vi "PID Proportional Control start.vi"(0 "Temp":dbl format="%.2f", 7 "Control Parameters":T1={"Setpoint"=50.0, "Control Bandwidth"=4.0, "Integral Time"=30.0, "Int\nON"=TRUE, "Derivative Tme"=0.5, "Der\nON"=TRUE, "Settle Bandwidth"=1.0, "Settle Time"=200.0} {"Settle Time" step=1.0; "Settle Bandwidth" step=0.01; "Derivative Tme" step=0.01; "Integral Time" step=1.0; "Control Bandwidth" step=0.1; "Setpoint" step=0.1}) -> (8 "Proportional Power":dbl format="%.2f")   [LabVIEW 2019]
doc: "Subvi\nThis does the proporianl part of the PID controller \n\nJuan Gamez\nP3600\nCSUSB"
uses:
  typedefs/PID control parameters.ctl
panel:
  # "PID\nProportional\nPower\nControl"
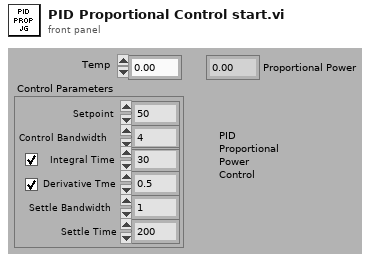
[diagram p1: front panel]
types:
  T1 = typedef "PID control parameters.ctl" = cluster{"Setpoint":dbl, "Control Bandwidth":dbl, "Integral Time":dbl, "Int\nON":bool, "Derivative Tme":dbl, "Der\nON":bool, "Settle Bandwidth":dbl, "Settle Time":dbl}
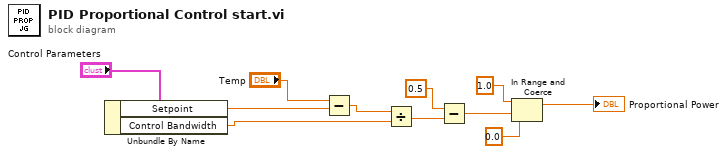
[diagram p0: block diagram]
diagram:
  n1 = Unbundle By Name("Control Parameters") -> ("Setpoint"=w10:dbl, "Control Bandwidth"=w8:dbl)
  n2 = Subtract(x="Temp", y=w10) -> (x-y=w7:dbl)
  n3 = Divide(x=w7, y=w8) -> (x/y=w6:dbl)
  n4 = Subtract(x=0.5, y=w6) -> (x-y=w4:dbl)
  n5 = In Range and Coerce(upper limit=1.0, x=w4, lower limit=0.0) -> (coerced(x)=→"Proportional Power":dbl)  [unwired: 1 out]
